vi "onDestroy.vi"(8 "error in (no error)":errorcluster, 11 "Client in":refnum<class "Client.lvclass">) -> (0 "error out":errorcluster, 3 "Client out":refnum<class "Client.lvclass">)   [LabVIEW 2013, in "MQTT Client.lvlib" / "Client.lvclass"]
uses:
  Client.lvclass
  <vilib>/LabVIEW Open Source Project/MQTT Connection/MQTT_Base/Base Class/MQTT_Base.lvclass
  Client.lvclass/Client.ctl
  Session.Client/Session.Client.lvclass
  <vilib>/LabVIEW Open Source Project/MQTT Connection/MQTT_Base/Session/Session.lvclass
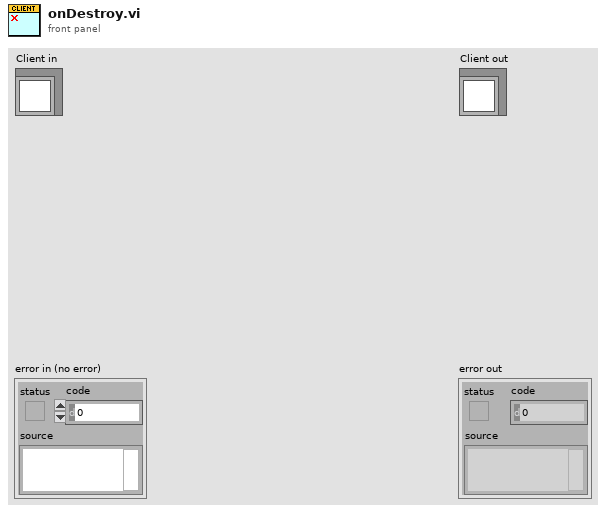
[diagram p1: front panel]
types:
  T1 = typedef "MQTT Client.lvlib/Client.lvclass/Public Events -- cluster.ctl" = cluster{"Connection Status":refnum<user-event>, "Connected":refnum<user-event>, "Application Message":refnum<user-event>}
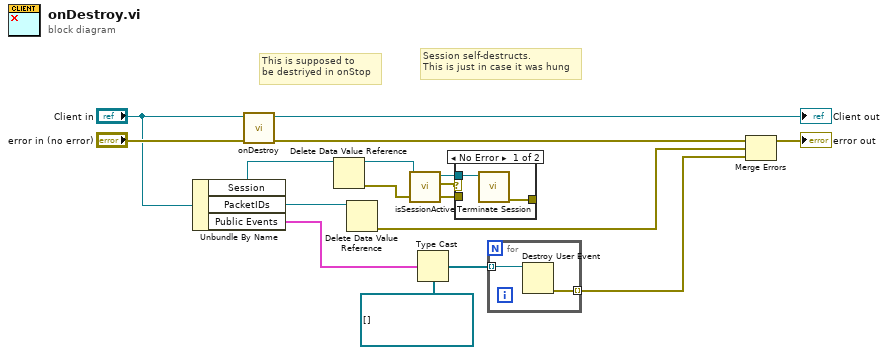
[diagram p0: block diagram]
diagram:
  # "This is supposed to\nbe destriyed in onStop"
  # "Session self-destructs.\nThis is just in case it was hung"
  n1 = Unbundle By Name("Client in") -> ("Session"=w3:refnum<data-value>, "PacketIDs"=w13:refnum<data-value>, "Public Events"=w7:T1)
  n2 = call-parent "onDestroy.vi"("error in (no error)"="error in (no error)", "MQTT_Base in"="Client in") -> ("error out"=w12:errorcluster, "MQTT_Base out"=→"Client out":refnum<class "Client.lvclass">)  [unwired: 8 in]
  n3 = Delete Data Value Reference(data value reference=w3) -> (data value=w2:refnum<class "Session.Client.lvclass">, error out=w1:errorcluster)  [unwired: 1 in]
  n4 = Delete Data Value Reference(data value reference=w13) -> (error out=w6:errorcluster)  [unwired: 1 in, 1 out]
  n5 = call <vilib>:"isSessionActive.vi"("Session in"=w2) -> ("error out"=w4:errorcluster, "Session out"=w5:refnum<class "Session.Client.lvclass">)  [unwired: 9 in]
  n6 = Type Cast(type=refnum<user-event>[] [], x=w7) -> (*(type *) &x=w9:refnum<user-event>[])
  n7 = case shown="No Error" w4 {
    tunnel: [w18 _] -> _
    tunnel: w5 -> [w17 _]
    tunnel: w1 -> [_ _]
    frame No Error {
      n8 = call <vilib>:"Terminate Session.vi"("Session in"=w17) -> ("error out"=w18:errorcluster)  [unwired: 8 in, 2 out]
    }
    frame Error {
    }
  }
  n9 = for {
    tunnel: w9 -> [w20] mode=indexing
    tunnel: [w19] -> w8 mode=indexing
    n10 = Destroy User Event(user event=w20) -> (error out=w19:errorcluster)  [unwired: 1 in]
  }
  n11 = Merge Errors(w12, w6, w8) -> (→"error out":errorcluster)
